vi "Destroy.vi"(8 "Error In":errorcluster, 11 "reference in":refnum<class "Measure and Stimulus Subsystems.lvclass">) -> (0 "Error Out":errorcluster, 3 "reference out":refnum<class "Measure and Stimulus Subsystems.lvclass">)   [LabVIEW 2023, in "HAL GOOP4.lvlib" / "Measure and Stimulus Subsystems.lvclass"]
uses:
  Measure and Stimulus Subsystems.lvclass
  Measure and Stimulus Subsystems.lvclass/Measure and Stimulus Subsystems.ctl
  Instrument Base/Instrument Base.lvclass
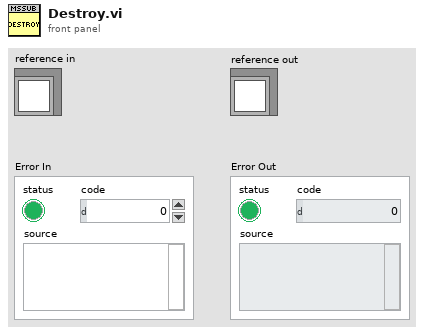
[diagram p1: front panel]
types:
  T1 = typedef "HAL GOOP4.lvlib/Measure and Stimulus Subsystems.lvclass/ObjectAttributes.ctl" = cluster{"Virt Instr":map{string, cluster{"Virtual Instrument Base":refnum<class "Virtual Instrument Base.lvclass">, "Phys Instr Channel":u8}}, "Phys Instr":map{string, cluster{"Instrument Base":refnum<class "Instrument Base.lvclass">, "Ref Count":u8}}}
  T2 = map{string, cluster{"Instrument Base":refnum<class "Instrument Base.lvclass">, "Ref Count":u8}}
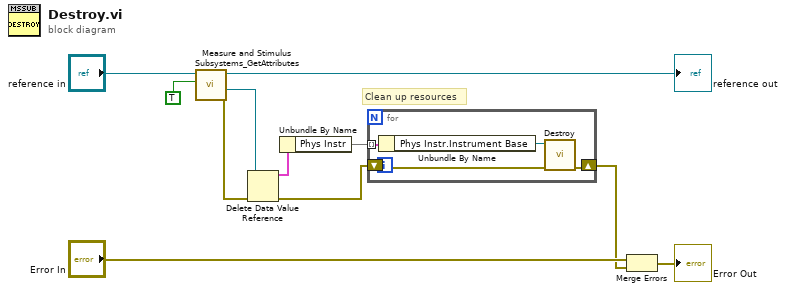
[diagram p0: block diagram]
diagram:
  # "Clean up resources"
  n1 = call "Measure and Stimulus Subsystems_GetAttributes.vi"("OnlyGetDvrReference(False)"=TRUE, "reference in"="reference in") -> ("Error Out"=w8:errorcluster, "DataRef"=w7:refnum<data-value>, "reference out"=→"reference out":refnum<class "Measure and Stimulus Subsystems.lvclass">)  [unwired: 6 in, 1 out]
  n2 = Delete Data Value Reference(data value reference=w7, error in=w8) -> (data value=w4:T1, error out=w2:errorcluster)
  n3 = Unbundle By Name(w4) -> ("Phys Instr"=w3:T2)
  n4 = for {
    tunnel: w3 -> [w15] mode=indexing
    shift-right: [w13] -> w1
    shift-left: w2 -> [w12]
    n5 = Unbundle By Name(w15) -> ("Phys Instr.Instrument Base"=w14:refnum<class "Instrument Base.lvclass">)
    n6 = call-dynamic "Destroy.vi"("Error In"=w12, "reference in"=w14) -> ("Error Out"=w13:errorcluster)  [unwired: 8 in, 1 out]
  }
  n7 = Merge Errors("Error In", w1) -> (→"Error Out":errorcluster)
